vi "Cal load cell.vi"() -> ()   [LabVIEW 2018]
uses:
  <vilib>/ptbypt/NI_PtbyPt.lvlib
panel:
  in  "Stop Button":bool
  out "Mean measurement":dbl
  out "Load Cell, Knee Brace":dynamicdata(graph)
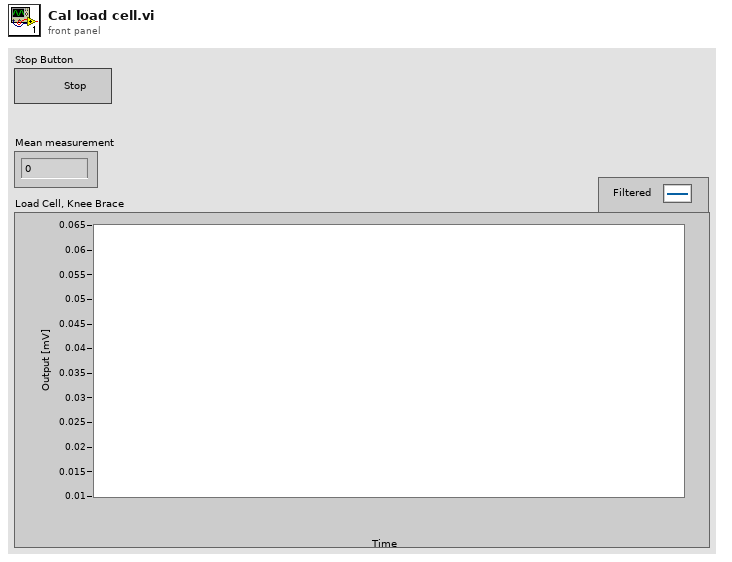
[diagram p1: front panel]
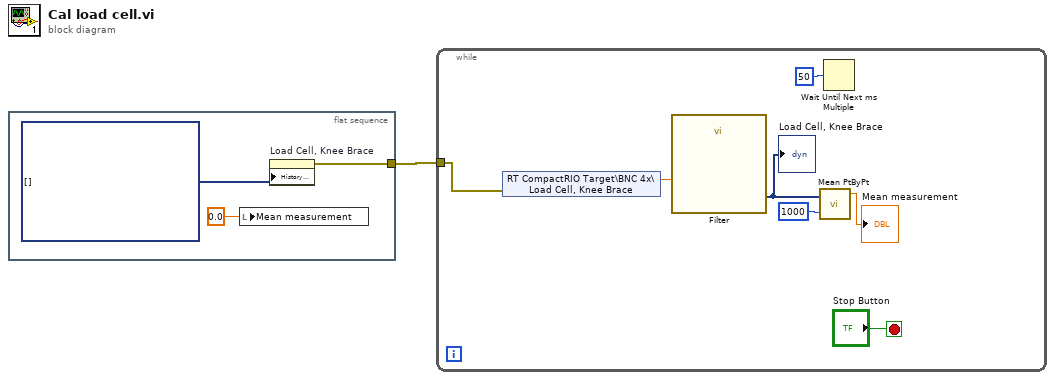
[diagram p0: block diagram]
diagram:
  n1 = flat-sequence {
    tunnel: [w4] -> w1
    frame #0 {
      n2 = local write "Mean measurement"(0.0 ("Mean measurement")) -> ()
      n3 = property on="Load Cell, Knee Brace" class="WFChart (strict)"("History Data"=dynamicdata[] []) -> (error out=w4:errorcluster)  [unwired: 2 in, 1 out]
    }
  }
  n4 = while {
    tunnel: w1 -> [w5]
    stop <- "Stop Button" stop-if-true
    n5 = shared-variable "RT CompactRIO Target\\BNC 4x\\Load Cell, Knee Brace"(error in=w5) -> (w9:dbl)  [unwired: 1 out]
    n6 = call "Filter"("Signal"=w9) -> ("Filtered Signal"=w7:dynamicdata)  [unwired: 9 in, 1 out]
    "Load Cell, Knee Brace" <- w7
    n7 = call <vilib>:"Mean PtByPt.vi"("x"=w7, "sample length"=1000) -> ("mean"=→"Mean measurement":dbl)  [unwired: 2 in, 1 out]
    n8 = Wait Until Next ms Multiple(millisecond multiple=u32 50) -> ()  [unwired: 1 out]
  }
